vi "popUPCrearNuevoObjetoRod.vi"() -> (2 "datosRod":T1, 3 "Listo Ingresar OD SteelGrade Lote":bool=TRUE)   [LabVIEW 2014]
panel:
  in  "textoFinCarga":string="Gracias por ingresar los datos del producto"
  in  "camposMedicion":string="camposMedicion"
  in  "idRod":string="numeroIDRod"
  in  "idImage":string="numIDImage"
  in  "idProducto":string="numIDProducto"
  in  "dateCreate":string="dateCreate"
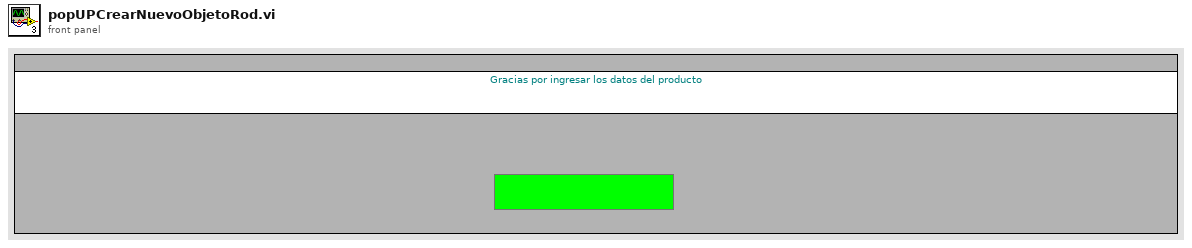
[diagram p1: front panel]
types:
  T1 = cluster{"idRod":string, "camposMedicion":string, "dateCreate":string, "idProducto":string, "idImage":string}
  T2 = enum8{"Enabled", "Disabled", "Disabled and Grayed Out"}
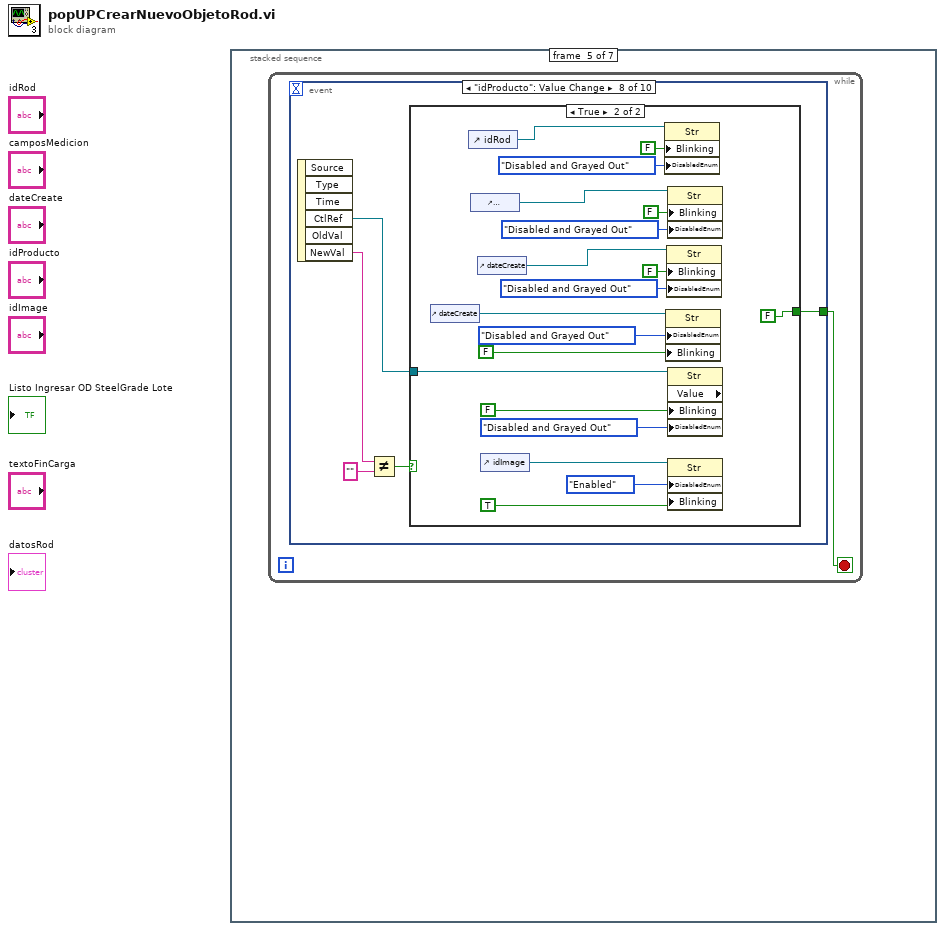
[diagram p0: block diagram]
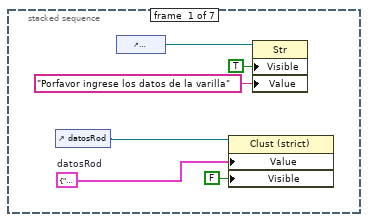
[diagram p2: hidden frame]
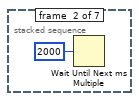
[diagram p3: hidden frame]
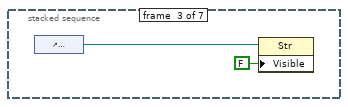
[diagram p4: hidden frame]
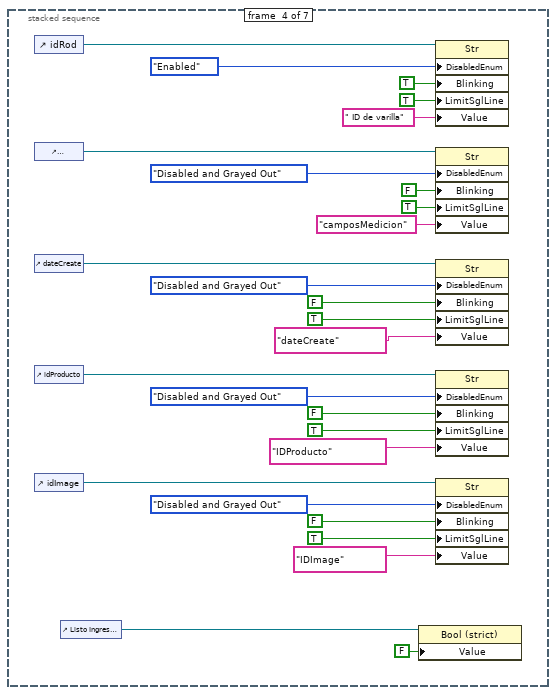
[diagram p5: hidden frame]
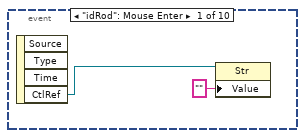
[diagram p6: hidden frame]
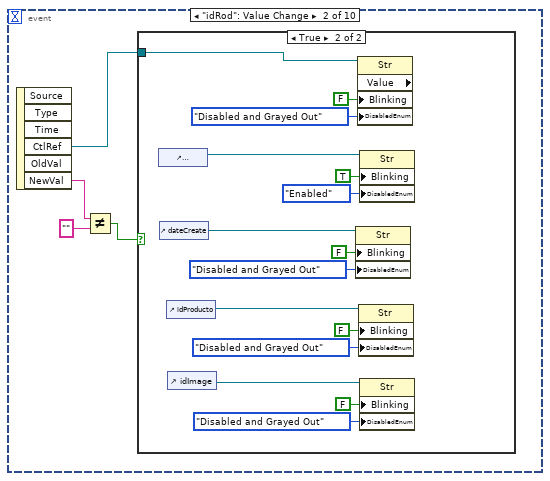
[diagram p7: hidden frame]
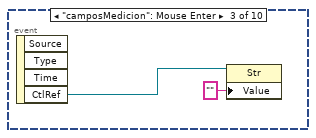
[diagram p9: hidden frame]
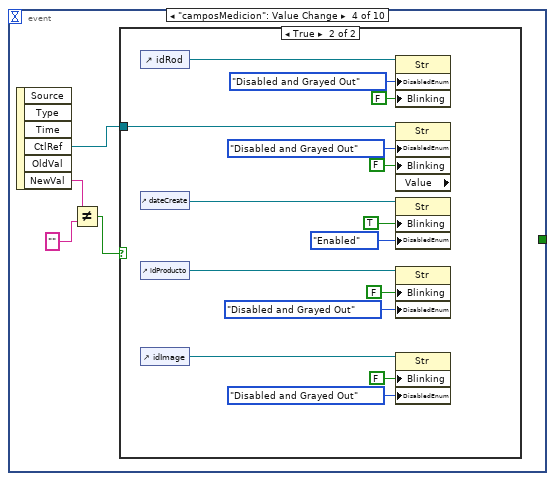
[diagram p10: hidden frame]
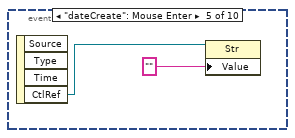
[diagram p12: hidden frame]
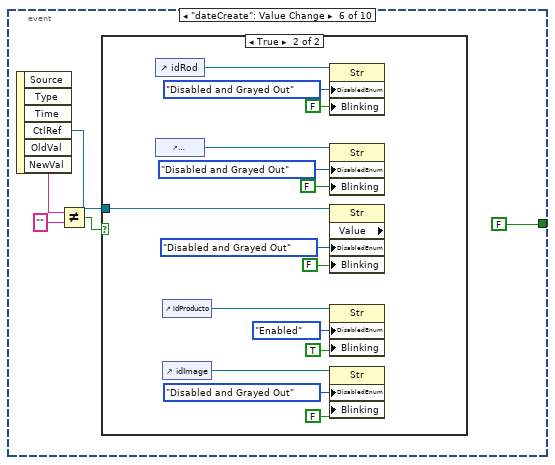
[diagram p13: hidden frame]
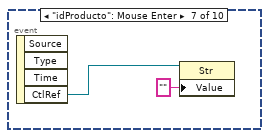
[diagram p15: hidden frame]
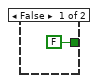
[diagram p16: hidden frame]
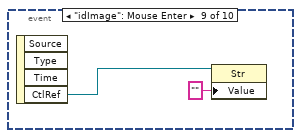
[diagram p17: hidden frame]
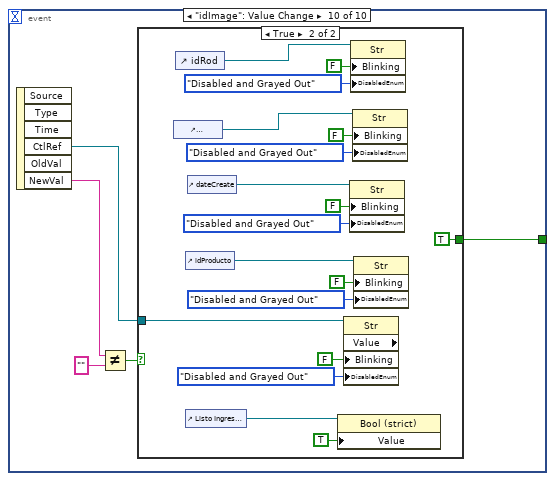
[diagram p18: hidden frame]
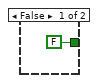
[diagram p19: hidden frame]
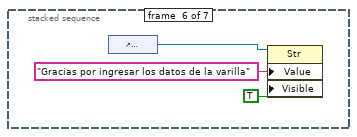
[diagram p20: hidden frame]
diagram:
  n1 = stacked-sequence {
    frame #0 {
      w1 = T1 {"idRod"="", "camposMedicion"="", "dateCreate"="", "idProducto"="", "idImage"=""}  # datosRod
      n2 = control-ref of="datosRod"() -> (w2:refnum<vi>)
      n3 = control-ref of="textoFinCarga"() -> (w6:refnum<vi>)
      n4 = property class="Clust (strict)"(reference=w2, "Value"=w1, "Visible"=FALSE) -> ()  [unwired: 1 in, 2 out]
      n5 = property class="Str"(reference=w6, "Visible"=TRUE, "Value"="Porfavor ingrese los datos de la varilla") -> ()  [unwired: 1 in, 2 out]
    }
    frame #1 {
      n6 = Wait Until Next ms Multiple(millisecond multiple=u32 2000) -> ()  [unwired: 1 out]
    }
    frame #2 {
      n7 = control-ref of="textoFinCarga"() -> (w9:refnum<vi>)
      n8 = property class="Str"(reference=w9, "Visible"=FALSE) -> ()  [unwired: 1 in, 2 out]
    }
    frame #3 {
      n9 = control-ref of="idRod"() -> (w19:refnum<vi>)
      n10 = control-ref of="camposMedicion"() -> (w14:refnum<vi>)
      n11 = control-ref of="dateCreate"() -> (w36:refnum<vi>)
      n12 = control-ref of="idProducto"() -> (w34:refnum<vi>)
      n13 = control-ref of="idImage"() -> (w32:refnum<vi>)
      n14 = control-ref of="Listo Ingresar OD SteelGrade Lote"() -> (w24:refnum<vi>)
      n15 = property class="Bool (strict)"(reference=w24, "Value"=FALSE) -> ()  [unwired: 1 in, 2 out]
      n16 = property class="Str"(reference=w19, "DisabledEnum"=T2."Enabled" ("Disabled"), "Blinking"=TRUE, "LimitSglLine"=TRUE ("Limit To Single Line?"), "Value"=" ID de varilla") -> ()  [unwired: 1 in, 2 out]
      n17 = property class="Str"(reference=w14, "DisabledEnum"=T2."Disabled and Grayed Out" ("Disabled"), "Blinking"=FALSE, "LimitSglLine"=TRUE ("Limit To Single Line?"), "Value"="camposMedicion") -> ()  [unwired: 1 in, 2 out]
      n18 = property class="Str"(reference=w36, "DisabledEnum"=T2."Disabled and Grayed Out" ("Disabled"), "Blinking"=FALSE, "LimitSglLine"=TRUE ("Limit To Single Line?"), "Value"="dateCreate") -> ()  [unwired: 1 in, 2 out]
      n19 = property class="Str"(reference=w34, "DisabledEnum"=T2."Disabled and Grayed Out" ("Disabled"), "Blinking"=FALSE, "LimitSglLine"=TRUE ("Limit To Single Line?"), "Value"="IDProducto") -> ()  [unwired: 1 in, 2 out]
      n20 = property class="Str"(reference=w32, "DisabledEnum"=T2."Disabled and Grayed Out" ("Disabled"), "Blinking"=FALSE, "LimitSglLine"=TRUE ("Limit To Single Line?"), "Value"="IDImage") -> ()  [unwired: 1 in, 2 out]
    }
    frame #4 {
      n21 = while {
        stop <- w37 stop-if-true
        n22 = event shown="[7] \"idProducto\": Value Change" {
          selector: _ -> [_ _ _ _ _ _ _ _ _ _]
          dyn-events: _ -> [_ _ _ _ _ _ _ _ _ _]
          timeout: _ -> [_ _ _ _ _ _ _ _ _ _]
          tunnel: [_ _ _ _ _ FALSE _ w107 _ w134] -> w37
          event "idRod": Mouse Enter {
            n23 = event-data() -> ("CtlRef"=w39:refnum<vi>)  [unwired: 1 in, 3 out]
            n24 = property class="Str"(reference=w39, "Value"="") -> ()  [unwired: 1 in, 2 out]
          }
          event "idRod": Value Change {
            n25 = event-data() -> ("CtlRef"=w40:refnum<vi>, "NewVal"=w43:string)  [unwired: 1 in, 4 out]
            n26 = Not Equal?(x=w43, y="") -> (x != y?=w41:bool)
            n27 = case shown="True" w41 {
              tunnel: w40 -> [_ w58]
              frame False {
              }
              frame True {
                n28 = control-ref of="camposMedicion"() -> (w55:refnum<vi>)
                n29 = control-ref of="dateCreate"() -> (w52:refnum<vi>)
                n30 = control-ref of="idProducto"() -> (w49:refnum<vi>)
                n31 = control-ref of="idImage"() -> (w46:refnum<vi>)
                n32 = property class="Str"(reference=w52, "Blinking"=FALSE, "DisabledEnum"=T2."Disabled and Grayed Out" ("Disabled")) -> ()  [unwired: 1 in, 2 out]
                n33 = property class="Str" props=["Value", "Blinking", "DisabledEnum"](reference=w58, "Blinking"=FALSE, "DisabledEnum"=T2."Disabled and Grayed Out" ("Disabled")) -> ()  [unwired: 1 in, 3 out]
                n34 = property class="Str"(reference=w49, "Blinking"=FALSE, "DisabledEnum"=T2."Disabled and Grayed Out" ("Disabled")) -> ()  [unwired: 1 in, 2 out]
                n35 = property class="Str"(reference=w55, "Blinking"=TRUE, "DisabledEnum"=T2."Enabled" ("Disabled")) -> ()  [unwired: 1 in, 2 out]
                n36 = property class="Str"(reference=w46, "Blinking"=FALSE, "DisabledEnum"=T2."Disabled and Grayed Out" ("Disabled")) -> ()  [unwired: 1 in, 2 out]
              }
            }
          }
          event "camposMedicion": Mouse Enter {
            n37 = event-data() -> ("CtlRef"=w60:refnum<vi>)  [unwired: 1 in, 3 out]
            n38 = property class="Str"(reference=w60, "Value"="") -> ()  [unwired: 1 in, 2 out]
          }
          event "camposMedicion": Value Change {
            n39 = event-data() -> ("CtlRef"=w61:refnum<vi>, "NewVal"=w64:string)  [unwired: 1 in, 4 out]
            n40 = Not Equal?(x=w64, y="") -> (x != y?=w62:bool)
            n41 = case shown="True" w62 {
              tunnel: w61 -> [_ w76]
              frame False {
              }
              frame True {
                n42 = control-ref of="idRod"() -> (w79:refnum<vi>)
                n43 = control-ref of="dateCreate"() -> (w73:refnum<vi>)
                n44 = control-ref of="idProducto"() -> (w70:refnum<vi>)
                n45 = control-ref of="idImage"() -> (w67:refnum<vi>)
                n46 = property class="Str"(reference=w79, "DisabledEnum"=T2."Disabled and Grayed Out" ("Disabled"), "Blinking"=FALSE) -> ()  [unwired: 1 in, 2 out]
                n47 = property class="Str" props=["DisabledEnum", "Blinking", "Value"](reference=w76, "DisabledEnum"=T2."Disabled and Grayed Out" ("Disabled"), "Blinking"=FALSE) -> ()  [unwired: 1 in, 3 out]
                n48 = property class="Str"(reference=w73, "Blinking"=TRUE, "DisabledEnum"=T2."Enabled" ("Disabled")) -> ()  [unwired: 1 in, 2 out]
                n49 = property class="Str"(reference=w70, "Blinking"=FALSE, "DisabledEnum"=T2."Disabled and Grayed Out" ("Disabled")) -> ()  [unwired: 1 in, 2 out]
                n50 = property class="Str"(reference=w67, "Blinking"=FALSE, "DisabledEnum"=T2."Disabled and Grayed Out" ("Disabled")) -> ()  [unwired: 1 in, 2 out]
              }
            }
          }
          event "dateCreate": Mouse Enter {
            n51 = event-data() -> ("CtlRef"=w81:refnum<vi>)  [unwired: 1 in, 3 out]
            n52 = property class="Str"(reference=w81, "Value"="") -> ()  [unwired: 1 in, 2 out]
          }
          event "dateCreate": Value Change {
            n53 = event-data() -> ("CtlRef"=w86:refnum<vi>, "NewVal"=w83:string)  [unwired: 1 in, 4 out]
            n54 = Not Equal?(x=w83, y="") -> (x != y?=w84:bool)
            n55 = case shown="True" w84 {
              tunnel: w86 -> [_ w101]
              frame False {
              }
              frame True {
                n56 = control-ref of="idRod"() -> (w89:refnum<vi>)
                n57 = control-ref of="camposMedicion"() -> (w92:refnum<vi>)
                n58 = control-ref of="idProducto"() -> (w98:refnum<vi>)
                n59 = control-ref of="idImage"() -> (w95:refnum<vi>)
                n60 = property class="Str"(reference=w89, "DisabledEnum"=T2."Disabled and Grayed Out" ("Disabled"), "Blinking"=FALSE) -> ()  [unwired: 1 in, 2 out]
                n61 = property class="Str"(reference=w92, "DisabledEnum"=T2."Disabled and Grayed Out" ("Disabled"), "Blinking"=FALSE) -> ()  [unwired: 1 in, 2 out]
                n62 = property class="Str" props=["Value", "DisabledEnum", "Blinking"](reference=w101, "DisabledEnum"=T2."Disabled and Grayed Out" ("Disabled"), "Blinking"=FALSE) -> ()  [unwired: 1 in, 3 out]
                n63 = property class="Str"(reference=w98, "DisabledEnum"=T2."Enabled" ("Disabled"), "Blinking"=TRUE) -> ()  [unwired: 1 in, 2 out]
                n64 = property class="Str"(reference=w95, "DisabledEnum"=T2."Disabled and Grayed Out" ("Disabled"), "Blinking"=FALSE) -> ()  [unwired: 1 in, 2 out]
              }
            }
          }
          event "idProducto": Mouse Enter {
            n65 = event-data() -> ("CtlRef"=w103:refnum<vi>)  [unwired: 1 in, 3 out]
            n66 = property class="Str"(reference=w103, "Value"="") -> ()  [unwired: 1 in, 2 out]
          }
          event "idProducto": Value Change {
            n67 = event-data() -> ("CtlRef"=w108:refnum<vi>, "NewVal"=w106:string)  [unwired: 1 in, 4 out]
            n68 = Not Equal?(x=w106, y="") -> (x != y?=w104:bool)
            n69 = case shown="True" w104 {
              tunnel: w108 -> [_ w128]
              tunnel: [FALSE FALSE] -> w107
              frame False {
              }
              frame True {
                n70 = control-ref of="dateCreate"() -> (w112:refnum<vi>)
                n71 = control-ref of="idRod"() -> (w115:refnum<vi>)
                n72 = control-ref of="camposMedicion"() -> (w120:refnum<vi>)
                n73 = control-ref of="dateCreate"() -> (w121:refnum<vi>)
                n74 = control-ref of="idImage"() -> (w126:refnum<vi>)
                n75 = property class="Str"(reference=w115, "Blinking"=FALSE, "DisabledEnum"=T2."Disabled and Grayed Out" ("Disabled")) -> ()  [unwired: 1 in, 2 out]
                n76 = property class="Str"(reference=w112, "DisabledEnum"=T2."Disabled and Grayed Out" ("Disabled"), "Blinking"=FALSE) -> ()  [unwired: 1 in, 2 out]
                n77 = property class="Str"(reference=w121, "Blinking"=FALSE, "DisabledEnum"=T2."Disabled and Grayed Out" ("Disabled")) -> ()  [unwired: 1 in, 2 out]
                n78 = property class="Str"(reference=w120, "Blinking"=FALSE, "DisabledEnum"=T2."Disabled and Grayed Out" ("Disabled")) -> ()  [unwired: 1 in, 2 out]
                n79 = property class="Str" props=["Value", "Blinking", "DisabledEnum"](reference=w128, "Blinking"=FALSE, "DisabledEnum"=T2."Disabled and Grayed Out" ("Disabled")) -> ()  [unwired: 1 in, 3 out]
                n80 = property class="Str"(reference=w126, "DisabledEnum"=T2."Enabled" ("Disabled"), "Blinking"=TRUE) -> ()  [unwired: 1 in, 2 out]
              }
            }
          }
          event "idImage": Mouse Enter {
            n81 = event-data() -> ("CtlRef"=w130:refnum<vi>)  [unwired: 1 in, 3 out]
            n82 = property class="Str"(reference=w130, "Value"="") -> ()  [unwired: 1 in, 2 out]
          }
          event "idImage": Value Change {
            n83 = event-data() -> ("CtlRef"=w135:refnum<vi>, "NewVal"=w133:string)  [unwired: 1 in, 4 out]
            n84 = Not Equal?(x=w133, y="") -> (x != y?=w132:bool)
            n85 = case shown="True" w132 {
              tunnel: w135 -> [_ w154]
              tunnel: [FALSE TRUE] -> w134
              frame False {
              }
              frame True {
                n86 = control-ref of="camposMedicion"() -> (w142:refnum<vi>)
                n87 = control-ref of="idRod"() -> (w139:refnum<vi>)
                n88 = control-ref of="idProducto"() -> (w147:refnum<vi>)
                n89 = control-ref of="Listo Ingresar OD SteelGrade Lote"() -> (w144:refnum<vi>)
                n90 = control-ref of="dateCreate"() -> (w150:refnum<vi>)
                n91 = property class="Bool (strict)"(reference=w144, "Value"=TRUE) -> ()  [unwired: 1 in, 2 out]
                n92 = property class="Str" props=["Value", "Blinking", "DisabledEnum"](reference=w154, "Blinking"=FALSE, "DisabledEnum"=T2."Disabled and Grayed Out" ("Disabled")) -> ()  [unwired: 1 in, 3 out]
                n93 = property class="Str"(reference=w150, "Blinking"=FALSE, "DisabledEnum"=T2."Disabled and Grayed Out" ("Disabled")) -> ()  [unwired: 1 in, 2 out]
                n94 = property class="Str"(reference=w139, "Blinking"=FALSE, "DisabledEnum"=T2."Disabled and Grayed Out" ("Disabled")) -> ()  [unwired: 1 in, 2 out]
                n95 = property class="Str"(reference=w142, "Blinking"=FALSE, "DisabledEnum"=T2."Disabled and Grayed Out" ("Disabled")) -> ()  [unwired: 1 in, 2 out]
                n96 = property class="Str"(reference=w147, "Blinking"=FALSE, "DisabledEnum"=T2."Disabled and Grayed Out" ("Disabled")) -> ()  [unwired: 1 in, 2 out]
              }
            }
          }
        }
      }
    }
    frame #5 {
      n97 = control-ref of="textoFinCarga"() -> (w157:refnum<vi>)
      n98 = property class="Str"(reference=w157, "Value"="Gracias por ingresar los datos de la varilla", "Visible"=TRUE) -> ()  [unwired: 1 in, 2 out]
    }
    frame #6 {
      w165 = T1 {"idRod"="", "camposMedicion"="", "dateCreate"="", "idProducto"="", "idImage"=""}  # datosRod
      n99 = control-ref of="idRod"() -> (w164:refnum<vi>)
      n100 = control-ref of="camposMedicion"() -> (w163:refnum<vi>)
      n101 = control-ref of="dateCreate"() -> (w170:refnum<vi>)
      n102 = control-ref of="idProducto"() -> (w169:refnum<vi>)
      n103 = control-ref of="idImage"() -> (w168:refnum<vi>)
      n104 = property class="Str"(reference=w164) -> ("Value"=w162:string)  [unwired: 1 in, 2 out]
      n105 = property class="Str"(reference=w163) -> ("Value"=w161:string)  [unwired: 1 in, 2 out]
      n106 = property class="Str"(reference=w170) -> ("Value"=w160:string)  [unwired: 1 in, 2 out]
      n107 = property class="Str"(reference=w169) -> ("Value"=w159:string)  [unwired: 1 in, 2 out]
      n108 = property class="Str"(reference=w168) -> ("Value"=w158:string)  [unwired: 1 in, 2 out]
      n109 = Wait Until Next ms Multiple(millisecond multiple=u32 2000) -> ()  [unwired: 1 out]
      n110 = Bundle(cluster=w165, "idRod"=w162, "camposMedicion"=w161, "dateCreate"=w160, "idProducto"=w159, "idImage"=w158) -> (w167:T1)
      n111 = control-ref of="datosRod"() -> (w166:refnum<vi>)
      n112 = property class="Clust (strict)"(reference=w166, "Value"=w167) -> ()  [unwired: 1 in, 2 out]
    }
  }
